vi "Uninit 1.vi"(2 "Container State":T1, 3 "Display State":T2) -> ()   [LabVIEW 2013, in "XControl 1.xctl"]
uses:
  XControl 1.xctl
  State 1.ctl
  <vilib>/_xctls/Container State.ctl
  <vilib>/_xctls/XControlSupport.lvlib
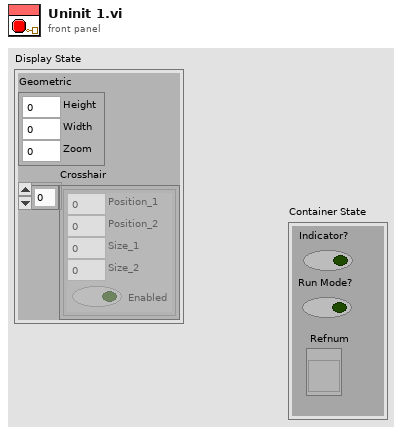
[diagram p1: front panel]
types:
  T1 = typedef "XControlSupport.lvlib/Container State.ctl" = cluster{"Indicator?":bool, "Run Mode?":bool, " Refnum":refnum<vi>}
  T2 = typedef "XControl 1.xctl/State 1.ctl" = cluster{"Geometric":cluster{"Height":dbl, "Width":dbl, "Zoom":dbl}, "Crosshair":cluster{"Position_1":dbl, "Position_2":dbl, "Size_1":dbl, "Size_2":dbl, "Enabled":bool}[]}
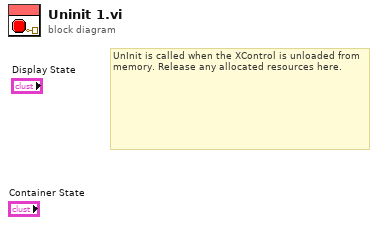
[diagram p0: block diagram]
diagram:
  # "UnInit is called when the XControl is unloaded from memory. Release any allocated resources here."
